vi "Compression with Wavelet (lossy).vi"() -> ()   [LabVIEW 2023]
doc: "This example shows the application of the discrete wavelet transform (DWT) in image compression.\n\nThe DWT transforms an image into wavelet coefficients. The wavelet coefficients have most values close to zero. After quantizing the wavelet coefficients, you can set most of the coefficients to zero. So you can use entropy-based encoding techniques to reduce the bit rate of the wavelet coefficients and achieve image compression.\n\nThis example uses the WA Discrete Wavelet Transform VI to transform an image into wavelet coefficients and simulates the quantization for the wavelet coefficients. From the quantized wavelet coefficients, this example reconstructs the image using the WA Inverse Discrete Wavelet Transform VI and computes the peak signal to noise ratio (PSNR) of the reconstructed image. In real-world image compression applications, you achieve compression by using entropy-based encoding techniques such as the Huffman coding to encode the quantized wavelet coefficients.\n\n<b>Instructions:</b>\n1) Run this VI.\n2) Change the number of <b>Bits</b> to quantize the wavelet transform and observe the <b>PSNR (dB)</b> of the image."
uses:
  Images/_Images.ctl
  <vilib>/addons/Wavelet Analysis/discrete wavelet transform.llb/WA 2D Discrete Wavelet Transform.vi
  <vilib>/addons/Wavelet Analysis/discrete wavelet transform.llb/WA Inverse 2D Discrete Wavelet Transform.vi
  <vilib>/addons/_Advanced Signal Processing/NI_AdvSigProcWA.lvlib
panel:
  in  "Image":T1=enum."Battery1"
  out "min diff":dbl
  out "max diff":dbl
  out "MSE":dbl
  out "Difference Image":T2(plugin-control)
  out "Reconstructed Image":T2(plugin-control)
  out "Original Image":T2(plugin-control)
  out "PSNR (dB)":dbl
  in  "Bits":i32=8 min=1 max=64
  in  "Wavelet":u16(ring) items=["db02"=0, "db03"=1, "db04"=2, "db05"=3, "db06"=4, "db07"=5, "db08"=6, "db09"=7, "db10"=8, "db11"=9, "db12"=10, "db13"=11, "db14"=12, "Haar"=13, "bior1_3"=14, "bior1_5"=15, "bior2_2"=16, "bior2_4"=17, "bior2_6"=18, "bior2_8"=19, "bior3_1"=20, "bior3_3"=21, "bior3_5"=22, "bior3_7"=23, "bior3_9"=24, "bior4_4 (FBI)"=25, "bior5_5"=38, "bior6_8"=39, "coif1"=26, "coif2"=27, "coif3"=28, "coif4"=29, "coif5"=30, "sym2"=31, "sym3"=32, "sym4"=33, "sym5"=34, "sym6"=35, "sym7"=36, "sym8"=37]
  in  "Levels":i32=8
  # "Discrete Wavelet Transform (DWT) - lossy image compression.\nAdvanced Signal Processing Toolkit is required"
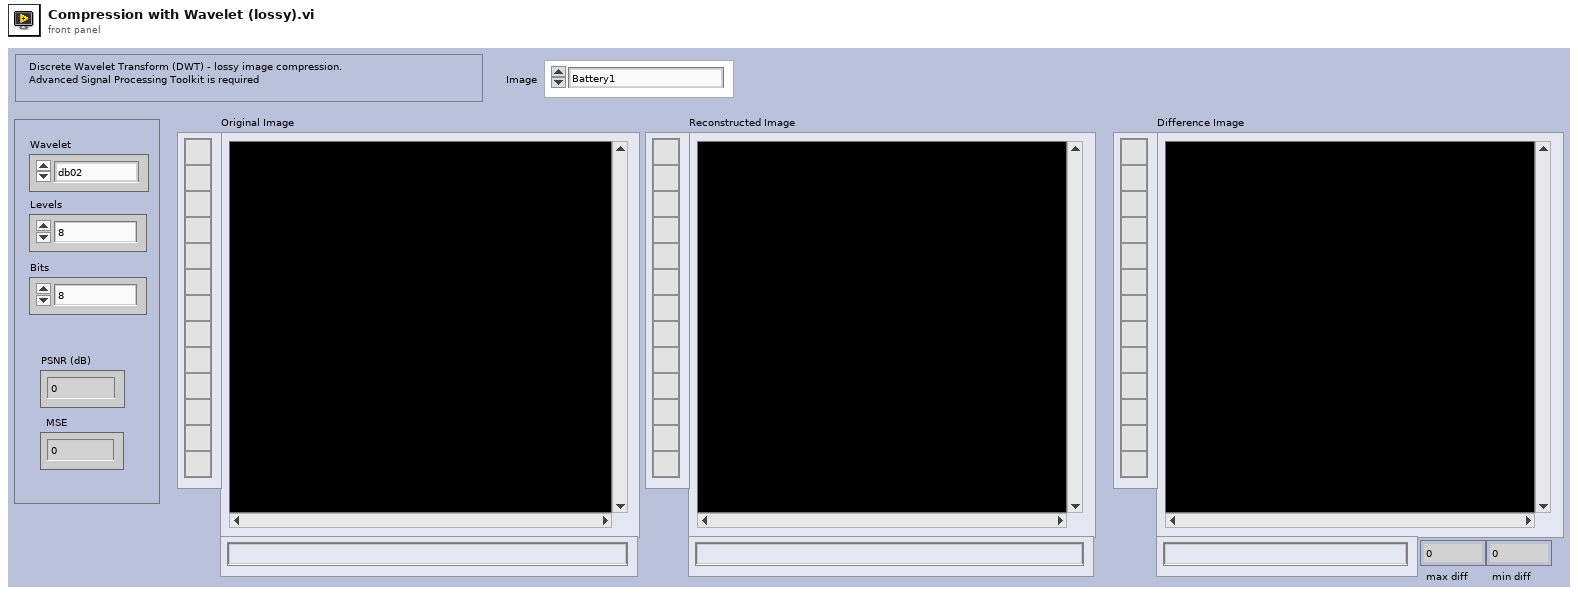
[diagram p1: front panel]
types:
  T1 = typedef "_Images.ctl" = enum16{"Balls2", "Battery1", "Battery2", "Connector1", "Subwoofer1", "Subwoofer2", "Subwoofer3", "Subwoofer4", "Hase1", "Lamp1", "Lamp2", "Mouse1", "PhotoLens1", "Po1", "PowerSupply1", "Router", "--- Step Wedges ---", "Stepwedge1", "Stepwedge2", "Stepwedge3", "--- Fusion ---", "Fusion160kV", "Fusion2-120kV", "Fusion2-320kV", "Fusion300kV", "FusionPart1-120kV", "FusionPart1-180kV", "--- PART 01 ---", "Part1", "Part2", "Part3", "Part4", "Part5", "Part6", "Part7", "Part8", "--- Different Integrations ---", "Step2737-02Int", "Step2737-04Int", "Step2737-08Int", "Step2737-16Int", "Step2737-32Int", "Step2737-64Int"}
  T2 = typedef "IMAQ Image.ctl" = refnum<image>
  T3 = typedef "Image Type" = u32
  T4 = cluster{"low_low":dbl[][], "low_high":dbl[][], "high_low":dbl[][], "high_high":dbl[][]}[]
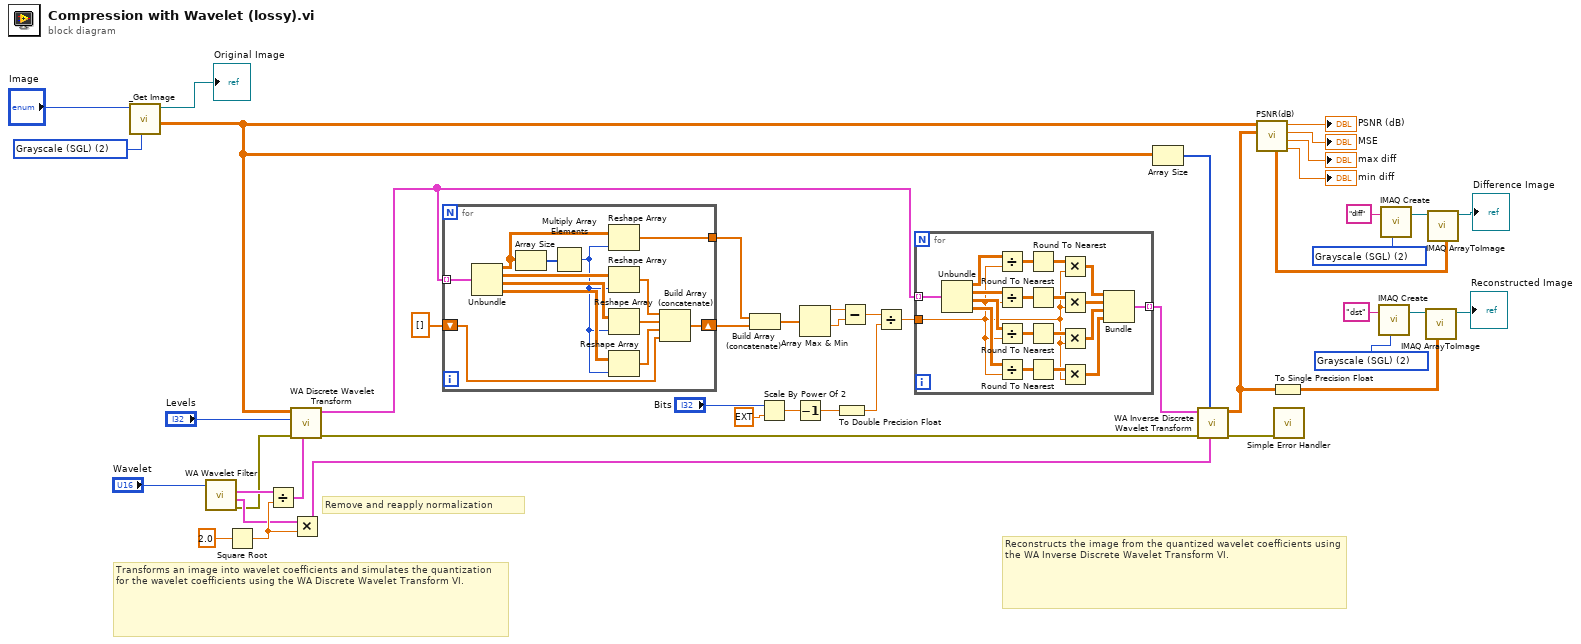
[diagram p0: block diagram]
diagram:
  w6 = T3 2 items=["Grayscale (U8)", "Grayscale (I16)", "Grayscale (SGL)", "Complex (CSG)", "RGB (U32)", "HSL (U32)", "RGB (U64)", "Grayscale (U16)"] ("Image Type")
  w29 = T3 2 items=["Grayscale (U8)", "Grayscale (I16)", "Grayscale (SGL)", "Complex (CSG)", "RGB (U32)", "HSL (U32)", "RGB (U64)", "Grayscale (U16)"] ("Image Type (U16)")
  w31 = T3 2 items=["Grayscale (U8)", "Grayscale (I16)", "Grayscale (SGL)", "Complex (CSG)", "RGB (U32)", "HSL (U32)", "RGB (U64)", "Grayscale (U16)"] ("Image Type")
  # "Remove and reapply normalization"
  # "Reconstructs the image from the quantized wavelet coefficients using the WA Inverse Discrete Wavelet Transform VI."
  # "Transforms an image into wavelet coefficients and simulates the quantization for the wavelet coefficients using the WA Discrete Wavelet Transform VI."
  n1 = call "_Get Image.vi"("Image Type (U16)"=w29, "Image"="Image") -> ("Image Pixels (Float)"=w28:dbl[][], "Image Out"=→"Original Image":T2)  [unwired: 6 in, 2 out]
  n2 = call <vilib>:"WA Wavelet Filter.vi"("wavelet"="Wavelet") -> ("error out"=w36:errorcluster, "synthesis filters"=w37:cluster{"lowpass":dbl[], "highpass":dbl[]}, "analysis filters"=w43:cluster{"lowpass":dbl[], "highpass":dbl[]})  [unwired: 3 in, 5 out]
  n3 = Square Root(x=2.0) -> (sqrt(x)=w38:dbl)
  n4 = Divide(x=w43, y=w38) -> (x/y=w40:cluster{"lowpass":dbl[], "highpass":dbl[]})
  n5 = call-poly <vilib>:"WA Discrete Wavelet Transform.vi"("analysis filters"=w40, "error in (no error)"=w36, "levels"="Levels", "signal"=w28) -> ("error out"=w35:errorcluster, "DWT coef"=w11:T4)  [unwired: 1 in, 5 out]
  n6 = Multiply(x=w37, y=w38) -> (x*y=w39:cluster{"lowpass":dbl[], "highpass":dbl[]})
  n7 = for {
    tunnel: w11 -> [w59] mode=indexing
    tunnel: [w53] -> w22
    shift-right: [w52] -> w23
    shift-left: dbl[] [] -> [w50]
    n8 = Unbundle(w59) -> ("low_low"=w58:dbl[][], "low_high"=w56:dbl[][], "high_low"=w55:dbl[][], "high_high"=w54:dbl[][])
    n9 = Array Size(array=w58) -> (size(s)=w57:i32[])
    n10 = Multiply Array Elements(1:w57) -> (0:w47:i32)
    n11 = Reshape Array(w58, w47) -> (w53:dbl[])
    n12 = Reshape Array(w56, w47) -> (w49:dbl[])
    n13 = Reshape Array(w55, w47) -> (w48:dbl[])
    n14 = Reshape Array(w54, w47) -> (w51:dbl[])
    n15 = Build Array (concatenate)(w49, w48, w51, w50) -> (w52:dbl[])
  }
  n16 = Build Array (concatenate)(w22, w23) -> (w13:dbl[])
  n17 = Scale By Power Of 2(n="Bits", x=ext 1.0) -> (x*2^n=w18:ext)
  n18 = Decrement(x=w18) -> (x-1=w19:ext)
  n19 = Array Max & Min(array=w13) -> (max value=w14:dbl, min value=w15:dbl)  [unwired: 2 out]
  n20 = To Double Precision Float(number=w19) -> (double precision float=w20:dbl)
  n21 = Subtract(x=w14, y=w15) -> (x-y=w16:dbl)
  n22 = Divide(x=w16, y=w20) -> (x/y=w12:dbl)
  n23 = for {
    tunnel: w12 -> [w65]
    tunnel: w11 -> [w78] mode=indexing
    tunnel: [w60] -> w9 mode=indexing
    n24 = Unbundle(w78) -> ("low_low"=w77:dbl[][], "low_high"=w68:dbl[][], "high_low"=w67:dbl[][], "high_high"=w66:dbl[][])
    n25 = Divide(x=w77, y=w65) -> (x/y=w76:dbl[][])
    n26 = Divide(x=w68, y=w65) -> (x/y=w73:dbl[][])
    n27 = Divide(x=w67, y=w65) -> (x/y=w72:dbl[][])
    n28 = Divide(x=w66, y=w65) -> (x/y=w69:dbl[][])
    n29 = Round To Nearest(number=w76) -> (nearest integer value=w75:dbl[][])
    n30 = Round To Nearest(number=w73) -> (nearest integer value=w74:dbl[][])
    n31 = Round To Nearest(number=w72) -> (nearest integer value=w71:dbl[][])
    n32 = Round To Nearest(number=w69) -> (nearest integer value=w70:dbl[][])
    n33 = Multiply(x=w75, y=w65) -> (x*y=w63:dbl[][])
    n34 = Multiply(x=w74, y=w65) -> (x*y=w64:dbl[][])
    n35 = Multiply(x=w71, y=w65) -> (x*y=w62:dbl[][])
    n36 = Multiply(x=w70, y=w65) -> (x*y=w61:dbl[][])
    n37 = Bundle(w63, w64, w62, w61) -> (w60:cluster{dbl[][], dbl[][], dbl[][], dbl[][]})  [unwired: 1 out]
  }
  n38 = Array Size(array=w28) -> (size(s)=w44:i32[])
  n39 = call-poly <vilib>:"WA Inverse Discrete Wavelet Transform.vi"("synthesis filters"=w39, "size"=w44, "error in (no error)"=w35, "DWT coef"=w9) -> ("error out"=w46:errorcluster, "signal"=w27:dbl[][])  [unwired: 1 in, 5 out]
  n40 = call "PSNR(dB).vi"("Image Pixels (Float) 2"=w27, "Image Pixels (Float) 1"=w28) -> ("min diff"=→"min diff":dbl, "max diff"=→"max diff":dbl, "Mean Square Error (MSE)"=→"MSE":dbl, "PSNR (dB)"=→"PSNR (dB)":dbl, "Difference"=w4:sgl[][])  [unwired: 5 in]
  n41 = To Single Precision Float(number=w27) -> (single precision float=w26:sgl[][])
  n42 = call <vilib>:"Simple Error Handler.vi"("error in (no error)"=w46) -> ()  [unwired: 1 in, 8 out]
  n43 = call "IMAQ Create"("Image Name"="dst", "Image Type"=w31) -> ("New Image"=w30:T2)  [unwired: 3 in, 1 out]
  n44 = call "IMAQ Create"("Image Name"="diff", "Image Type"=w6) -> ("New Image"=w7:T2)  [unwired: 3 in, 1 out]
  n45 = call "IMAQ ArrayToImage"("Image Pixels (Float)"=w26, "Image"=w30) -> ("Image Out"=→"Reconstructed Image":T2)  [unwired: 8 in, 1 out]
  n46 = call "IMAQ ArrayToImage"("Image Pixels (Float)"=w4, "Image"=w7) -> ("Image Out"=→"Difference Image":T2)  [unwired: 8 in, 1 out]
